vi "Test DAQ.vi"() -> ()   [LabVIEW 2013]
uses:
  SLL DAQ Engine/Software/Source Code/Sub VIs/DAQ Engine/Controls/SLL DE DI Global Options.ctl
  SLL DAQ Engine/Software/Source Code/Sub VIs/DAQ Engine/Controls/SLL DE DAQ Global Options.ctl
  SLL DAQ Engine/Software/Source Code/Sub VIs/DAQ Engine/Controls/SLL DE DAQ Global Elements.ctl
panel:
  out "Digital Array Status":bool[](array[boolean])
  in  "stop":bool
  out "error out":errorcluster
  in  "error in (no error)":errorcluster
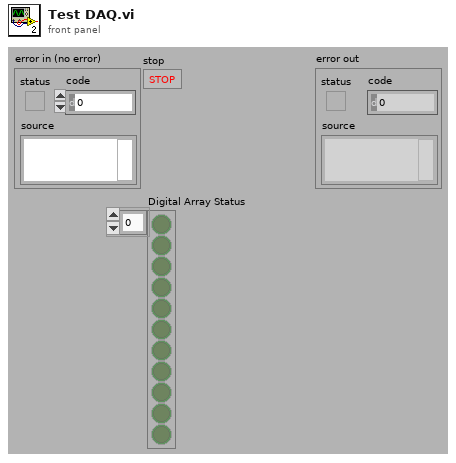
[diagram p1: front panel]
types:
  T1 = typedef "SLL DE DAQ Global Elements.ctl" = enum16{"AI Error", "AO Error", "DI Error", "DO Error", "AI Restart", "DI Restart", "AI Running", "AO Running", "DI Running", "DO Running", "DAQ Exit?"}
  T2 = typedef "SLL DE DAQ Global Options.ctl" = enum16{"Init", "Write 1", "Read 1", "Write Array", "Read Array", "Clear"}
  T3 = typedef "SLL DE DI Global Options.ctl" = enum16{"Init", "Write Line", "Write Array", "Read Line", "Read Array", "Read Full Status", "Write Full Status"}
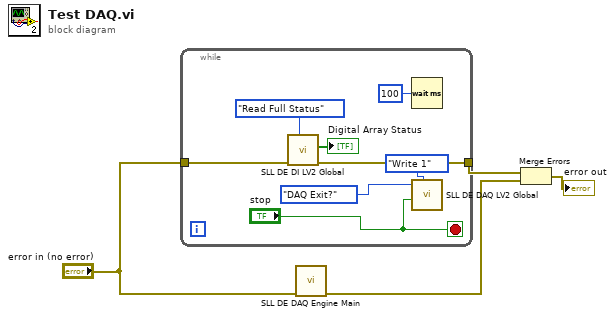
[diagram p0: block diagram]
diagram:
  n1 = while {
    tunnel: "error in (no error)" -> [w10]
    tunnel: [w9] -> w2
    stop <- "stop" stop-if-true
    n2 = call "SLL DE DI LV2 Global.vi"("Option"=SLL_DE_DI_Global_Options."Read Full Status", "error in (no error)"=w10) -> ("error out"=w9:errorcluster, "Digital Array Status"=→"Digital Array Status":bool[])  [unwired: 6 in, 2 out]
    n3 = Wait (ms)(milliseconds to wait=u32 100) -> ()  [unwired: 1 out]
    n4 = call "SLL DE DAQ LV2 Global.vi"("Option"=SLL_DE_DAQ_Global_Options."Write 1", "Status In"="stop", "Element"=SLL_DE_DAQ_Global_Elements."DAQ Exit?") -> ()  [unwired: 6 in, 3 out]
  }
  n5 = call "SLL DE DAQ Engine Main.vi"("error in (no error)"="error in (no error)") -> ("error out"=w3:errorcluster)  [unwired: 10 in]
  n6 = Merge Errors(w2, w3) -> (→"error out":errorcluster)
